vi "TB-Save Cal Signal.vi"(0 "Params":T1={"Low cutoff (kHz)"=0.0, "High cutoff (kHz)"=0.0, "Duration (min)"=0.0, "dB SPL"=100.0, "Waveform"=enum."Noise", "WAVfile"=path "", "refWav"=path "", "use mic correction"=FALSE, "micCorrFile"=path "", "Pistonphone Level (dB SPL)"=0.0, "Sampling rate (Hz)"=0.0, "Buffer length (s)"=0.0, "Stream mic"=FALSE, "Fine adjust"={"Max"=0.0, "Min"=0.0}, "Mic gain"=0.0, "atten"=0.0, "resol (Hz)"=0.0, "navgs"=0, "Allow Slack"=FALSE, "max starts"=0, "Freq (kHz)"=8.0, "Tma (s)"=0.0, "Streamed"=[], "Drive"="", "Speaker"="", "Mic"=""}, 2 "ID":string, 9 "Mic signal":dbl[](array[numeric])) -> (15 "error out":errorcluster)   [LabVIEW 2020]
uses:
  Typedefs/TB-Parameters.ctl
  <vilib>/sound2/lvsound2.llb/Sound Data Format.ctl
  <vilib>/sound2/lvsound2.llb/Sound File Write Open.vi
  <vilib>/sound2/lvsound2.llb/Sound File Write (DBL).vi
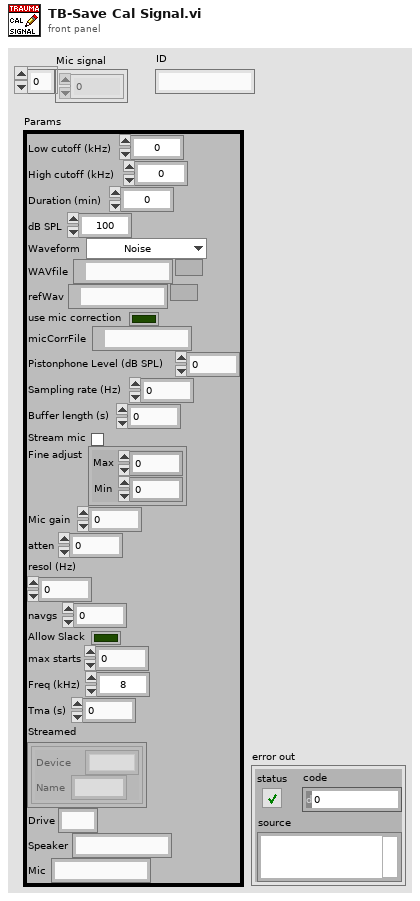
[diagram p1: front panel]
types:
  T1 = typedef "TB-Parameters.ctl" = cluster{"Low cutoff (kHz)":dbl, "High cutoff (kHz)":dbl, "Duration (min)":dbl, "dB SPL":dbl, "Waveform":enum16{"Noise", "File", "Tone"}, "WAVfile":path, "refWav":path, "use mic correction":bool, "micCorrFile":path, "Pistonphone Level (dB SPL)":dbl, "Sampling rate (Hz)":dbl, "Buffer length (s)":dbl, "Stream mic":bool, "Fine adjust":cluster{"Max":dbl, "Min":dbl}, "Mic gain":dbl, "atten":dbl, "resol (Hz)":dbl, "navgs":i32, "Allow Slack":bool, "max starts":i32, "Freq (kHz)":dbl, "Tma (s)":dbl, "Streamed":cluster{"Device":string, "Name":string}[], "Drive":string, "Speaker":string, "Mic":string}
  T2 = typedef "Sound Data Format.ctl" = cluster{"sample rate (S/s)":dbl, "number of channels":i32, "bits per sample":i32}
  T3 = typedef "Sound File Refnum.ctl" = refnum<file>
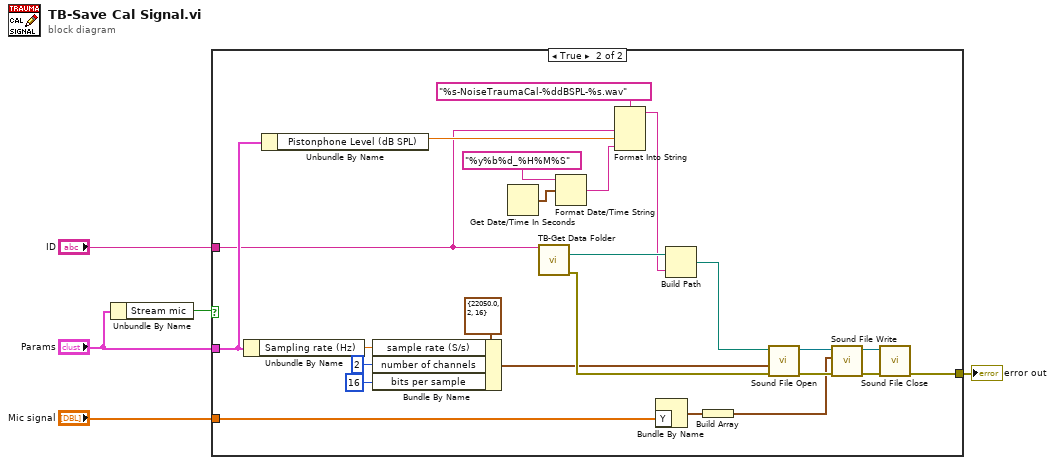
[diagram p0: block diagram]
diagram:
  n1 = Unbundle By Name("Params") -> ("Stream mic"=w5:bool)
  n2 = case shown="True" w5 {
    tunnel: "Params" -> [_ w9]
    tunnel: "ID" -> [_ w6]
    tunnel: "Mic signal" -> [_ w21]
    tunnel: [_ w7] -> w1
    frame False {
    }
    frame True {
      n3 = Unbundle By Name(w9) -> ("Sampling rate (Hz)"=w8:dbl)
      n4 = Unbundle By Name(w9) -> ("Pistonphone Level (dB SPL)"=w23:dbl)
      n5 = Bundle By Name(cluster=T2 {"sample rate (S/s)"=22050.0, "number of channels"=2, "bits per sample"=16} ("sound format"), "sample rate (S/s)"=w8, "number of channels"=2, "bits per sample"=16) -> (w12:T2)
      n6 = Get Date/Time In Seconds() -> (seconds since 1Jan1904=w26:timestamp)
      n7 = call "TB-Get Data Folder.vi"("ID"=w6) -> ("Data folder"=w29:path, "error out"=w15:errorcluster)  [unwired: 13 in]
      n8 = Format Date/Time String(time format string (%c)="%y%b%d_%H%M%S", seconds (now)=w26) -> (date/time string=w24:string)  [unwired: 1 in]
      n9 = Format Into String(format string="%s-NoiseTraumaCal-%ddBSPL-%s.wav", w6, w23, w24) -> (resulting string=w27:string)  [unwired: 2 in, 1 out]
      n10 = Bundle By Name("Y"=w21) -> (w22:waveform(dbl))  [unwired: 1 in]
      n11 = Build Path(base path=w29, name or relative path=w27) -> (appended path=w20:path)
      n12 = Build Array(w22) -> (w14:waveform(dbl)[])
      n13 = call-poly <vilib>:"Sound File Open.vi"("error in (no error)"=w15, "sound format"=w12, "path"=w20) -> ("error out"=w17:errorcluster, "sound file refnum"=w19:T3)  [unwired: 7 in]
      n14 = call-poly <vilib>:"Sound File Write.vi"("error in (no error)"=w17, "data"=w14, "sound file refnum"=w19) -> ("error out"=w16:errorcluster, "sound file refnum out"=w18:T3)  [unwired: 7 in]
      n15 = call <vilib>:"Sound File Close.vi"("error in (no error)"=w16, "sound file refnum"=w18) -> ("error out"=w7:errorcluster)  [unwired: 9 in]
    }
  }
  "error out" <- w1
